vi "sample.vi"() -> ()   [LabVIEW 2012]
uses:
  <vilib>/Utility/file.llb/Read From Spreadsheet File (I64).vi
panel:
  in  "Filter Width":i32
  out "Frequency":i64
  in  "Characterization Values":path
  out "Sample Value":dbl format="%#_4f"
  out "temp 4":dbl
  out "Strip Chart":dbl(graph)
  in  "Delay (ms)":u32(knob)=500 scale=0.0..2000.0
  in  "Sample File":path
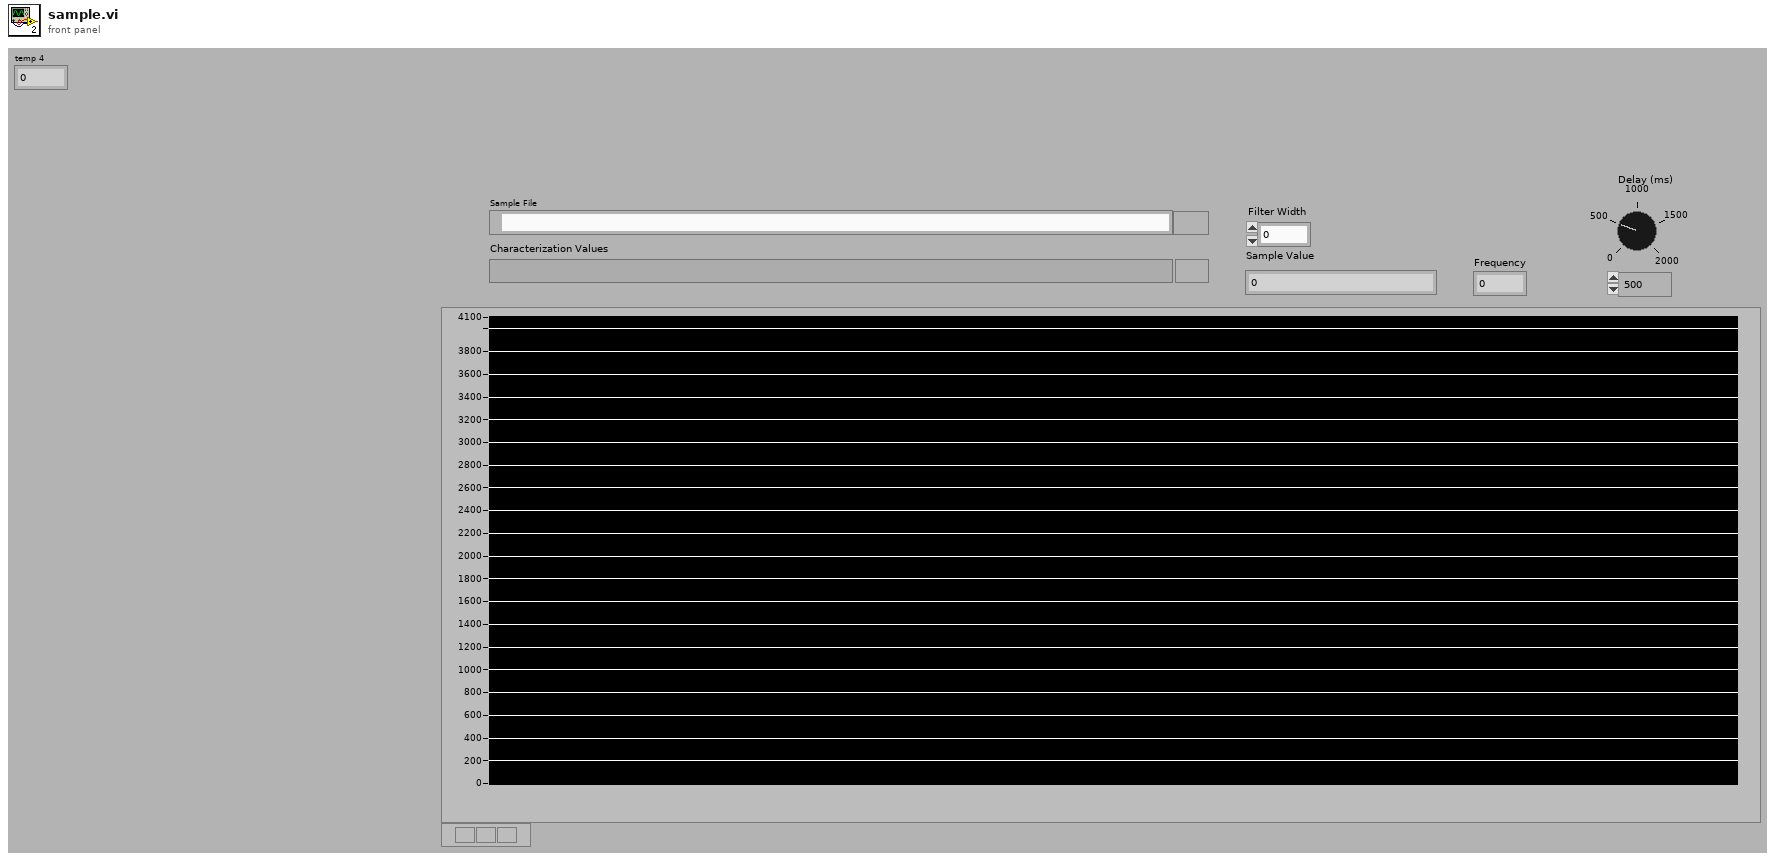
[diagram p1: front panel]
types:
  T1 = cluster{"second":i32, "minute":i32, "hour":i32, "day of month":i32, "month":i32, "year":i32, "day of week":i32, "day of year":i32, "is DST":i32}
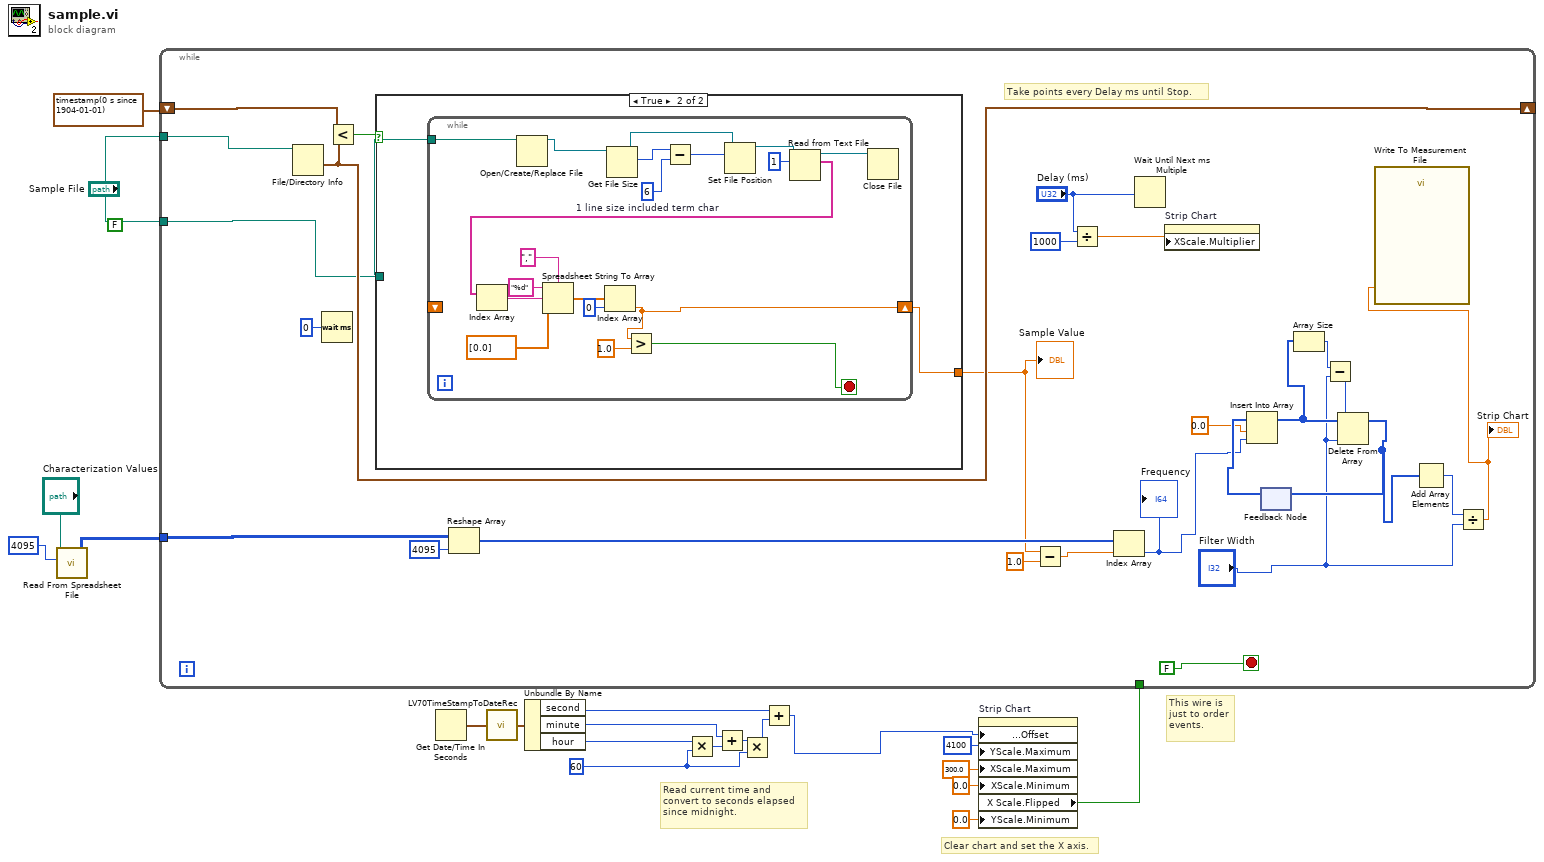
[diagram p0: block diagram]
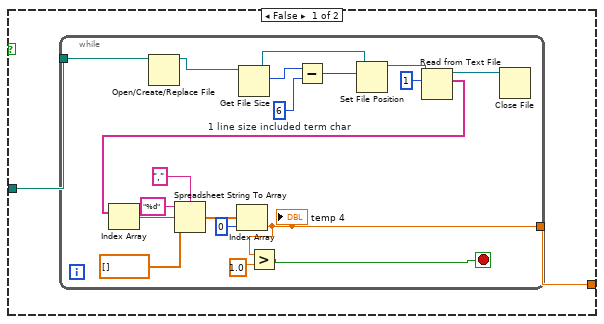
[diagram p2: hidden frame]
diagram:
  w9 = 60
  (unwired) FALSE ("disable buffering (F)")
  # "Read current time and\nconvert to seconds elapsed\nsince midnight."
  # "This wire is\njust to order\nevents."
  # "Clear chart and set the X axis."
  n1 = call-poly <vilib>:"Read From Spreadsheet File.vi"("number of rows (all:-1)"=4095, "file path (dialog if empty)"="Characterization Values") -> ("all rows"=w13:i64[][])  [unwired: 5 in, 4 out]
  n2 = Get Date/Time In Seconds() -> (seconds since 1Jan1904=w10:timestamp)
  n3 = call <vilib>:"LV70TimeStampToDateRec.vi"("time stamp"=w10) -> ("date time rec"=w2:T1)
  n4 = Unbundle By Name(w2) -> ("second"=w8:i32, "minute"=w5:i32, "hour"=w3:i32)
  n5 = Multiply(x=w3, y=w9) -> (x*y=w4:i32)
  n6 = Add(x=w5, y=w4) -> (x+y=w6:i32)
  n7 = Multiply(x=w6, y=w9) -> (x*y=w7:i32)
  n8 = Add(x=w8, y=w7) -> (x+y=w1:i32)
  n9 = property on="Strip Chart" class="WFChart (strict)"("X Scale.Offset and Multiplier:Offset"=w1, "YScale.Maximum"=4100, "XScale.Maximum"=300.0 ("X Scale.Range:Maximum"), "XScale.Minimum"=0.0 ("X Scale.Range:Minimum"), "YScale.Minimum"=0.0 ("Y Scale.Range:Maximum")) -> ("X Scale.Flipped"=w19:bool)  [unwired: 2 in, 2 out]
  n10 = while {
    tunnel: "Sample File" -> [w46]
    shift-right: [w44] -> _
    shift-left: timestamp(0 s since 1904-01-01) ("last mod") -> [w45]
    tunnel: w19 -> [_]
    tunnel: "Sample File" -> [w43]
    tunnel: w13 -> [w42]
    stop <- FALSE stop-if-true
    # "Take points every Delay ms until Stop."
    n11 = File/Directory Info(path=w46) -> (last mod=w44:timestamp)  [unwired: 1 in, 6 out]
    n12 = Wait (ms)(milliseconds to wait=u32 0) -> ()  [unwired: 1 out]
    n13 = Less?(x=w45, y=w44) -> (x < y?=w39:bool)
    n14 = case shown="True" w39 {
      tunnel: w43 -> [w48 w69]
      tunnel: [w47 w68] -> w25
      frame False {
        n15 = while {
          tunnel: [w49] -> w47
          tunnel: w48 -> [w53]
          stop <- w51 stop-if-true
          w60 = i64 6  # 1 line size included term char
          n16 = Open/Create/Replace File(file path (use dialog)=w53) -> (refnum out=w55:refnum<file>)  [unwired: 1 in, 6 out]
          n17 = Get File Size(file=w55) -> (refnum out=w58:refnum<file>, size (in bytes)=w61:i64)  [unwired: 1 in, 1 out]
          n18 = Subtract(x=w61, y=w60) -> (x-y=w59:i64)
          n19 = Set File Position(offset (in bytes) (0)=w59, refnum=w58) -> (refnum out=w56:refnum<file>)  [unwired: 1 in, 2 out]
          n20 = Read from Text File(file (use dialog)=w56, count=1) -> (refnum out=w52:refnum<file>, text=w54:string[])  [unwired: 1 in, 3 out]
          n21 = Index Array(array=w54) -> (element=w63:string)  [unwired: 1 in]
          n22 = Spreadsheet String To Array(delimiter (Tab)=",", format string="%d", spreadsheet string=w63, array type (2D Dbl)=dbl[] []) -> (array=w65:dbl[])
          n23 = Index Array(array=w65, index=0) -> (element=w49:dbl)
          "temp 4" <- w49
          n24 = Greater?(x=w49, y=1.0) -> (0:w51:bool)
          n25 = Close File(refnum=w52) -> ()  [unwired: 1 in, 2 out]
        }
      }
      frame True {
        n26 = while {
          tunnel: w69 -> [w74]
          shift-right: [w70] -> w68
          shift-left: _ -> [_]
          stop <- w72 stop-if-true
          w81 = i64 6  # 1 line size included term char
          n27 = Open/Create/Replace File(file path (use dialog)=w74) -> (refnum out=w76:refnum<file>)  [unwired: 1 in, 6 out]
          n28 = Get File Size(file=w76) -> (refnum out=w79:refnum<file>, size (in bytes)=w82:i64)  [unwired: 1 in, 1 out]
          n29 = Subtract(x=w82, y=w81) -> (x-y=w80:i64)
          n30 = Set File Position(offset (in bytes) (0)=w80, refnum=w79) -> (refnum out=w77:refnum<file>)  [unwired: 1 in, 2 out]
          n31 = Read from Text File(file (use dialog)=w77, count=1) -> (refnum out=w73:refnum<file>, text=w75:string[])  [unwired: 1 in, 3 out]
          n32 = Index Array(array=w75) -> (element=w84:string)  [unwired: 1 in]
          n33 = Spreadsheet String To Array(delimiter (Tab)=",", format string="%d", spreadsheet string=w84, array type (2D Dbl)=dbl[] [0.0]) -> (array=w86:dbl[])
          n34 = Index Array(array=w86, index=0) -> (element=w70:dbl)
          n35 = Greater?(x=w70, y=1.0) -> (0:w72:bool)
          n36 = Close File(refnum=w73) -> ()  [unwired: 1 in, 2 out]
        }
      }
    }
    "Sample Value" <- w25
    n37 = Reshape Array(w42, 4095 ("dimension size")) -> (w36:i64[])
    n38 = Subtract(x=w25, y=1.0) -> (x-y=w37:dbl)
    n39 = Divide(x="Delay (ms)", y=u32 1000) -> (x/y=w24:dbl)
    n40 = Index Array(array=w36, index=w37) -> (element=w30:i64)
    "Frequency" <- w30
    n41 = Wait Until Next ms Multiple(millisecond multiple="Delay (ms)") -> ()  [unwired: 1 out]
    n42 = property on="Strip Chart" class="WFChart (strict)"("XScale.Multiplier"=w24) -> ()  [unwired: 2 in, 2 out]
    n43 = feedback #1() -> (w32:i64[])  [unwired: 1 in]
    n44 = Insert Into Array(array=w32, index=0.0 ("new element/subarray"), new element=w30) -> (w28:i64[])
    n45 = Array Size(array=w28) -> (size(s)=w27:i32)
    n46 = Subtract(x=w27, y="Filter Width") -> (x-y=w26:i32)
    n47 = Delete From Array(array=w28, length=w26, index="Filter Width") -> (array with subset deleted=w29:i64[])  [unwired: 1 out]
    n48 = feedback-in #1(w29) -> ()
    n49 = Add Array Elements(numeric array=w29) -> (sum=w23:i64)
    n50 = Divide(x=w23, y="Filter Width") -> (x/y=w21:dbl)
    "Strip Chart" <- w21
    n51 = call "Write To Measurement File"("Signals"=w21) -> ()  [unwired: 16 in, 3 out]
  }
